vi "MeasureRMS.vi"(2 "Sampling Rate":dbl, 3 "# of Samples":dbl) -> (0 "Waveform Graph":dynamicdata(graph), 1 "RMS":dbl)   [LabVIEW 2015]
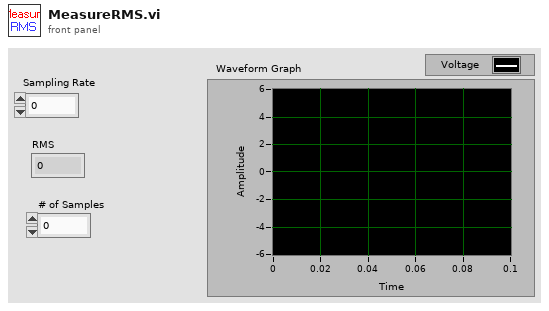
[diagram p1: front panel]
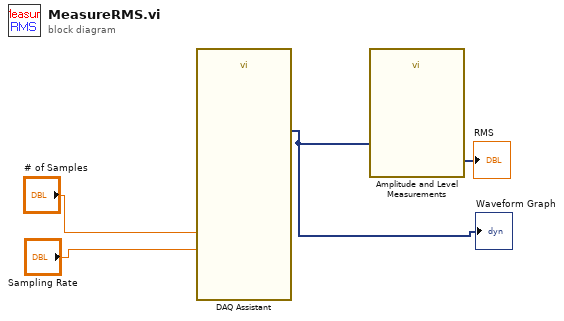
[diagram p0: block diagram]
diagram:
  n1 = call "DAQ Assistant"("rate"="Sampling Rate", "number of samples"="# of Samples") -> ("data"=w1:dynamicdata)  [unwired: 14 in, 3 out]
  "Waveform Graph" <- w1
  n2 = call "Amplitude and Level Measurements"("Signals"=w1) -> ("RMS"=→"RMS":dynamicdata)  [unwired: 13 in, 1 out]
